vi "RT.vi"() -> ()   [LabVIEW 2013]
uses:
  <vilib>/rvi/interface/nirviOpenFPGA/nirviOpenFPGA.xnode
  <vilib>/rvi/interface/nirviCloseFPGA/nirviCloseFPGA.xnode
  <vilib>/rvi/interface/nirviReadWriteControl/nirviReadWriteControl.xnode
  <vilib>/rvi/interface/Simulation/niFpgaSimulationCallBeginRW.vi
  <vilib>/rvi/errors/niLvFpgaAdjustHostInterfaceError.vi
  <vilib>/Utility/error.llb/Error Cluster From Error Code.vi
  FPGA Bitfiles/AudurLoadControl_FPGATarget_FPGA_+jw7eAiF5hA.lvbitx
  FPGA.vi
  <vilib>/FPGAPlugInAG/cRIO-9082/niLvFpga_Open_cRIO-9082.vi
  <vilib>/rvi/interface/common/dynamic/niFpgaDynamicAddResources.vi
  NiFpgaLv.dll
  <vilib>/FPGAPlugInAG/Dynamic/niLvFpga_Close_Dynamic.vi
panel:
  in  "Alpha":sgl
  in  "Scaling":sgl
  in  "Freq of Osc":sgl
  out "Monitoring Loop Period":u32
  out "Input Selection Loop Period":u32
  in  "Input pick":u16
  # "Input singal picking:\n0 Active Power \n1 Positive seq. volt A1\n2 Positive seq. volt A2\n3 Positive seq. current A1\n4 Positive seq. current A2\n5 Volt angle difference"
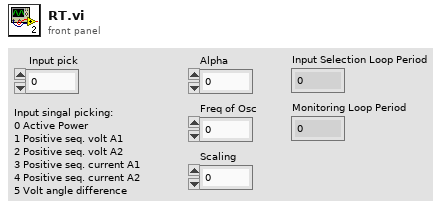
[diagram p1: front panel]
types:
  T1 = cluster{"Parameters":cluster{"Ts":sgl, "kappaav":sgl, "kappaph":sgl, "mu":sgl}}
  T2 = cluster{"Input signal":sgl, "Control signal":sgl, " Empty":sgl, " Empty":sgl}
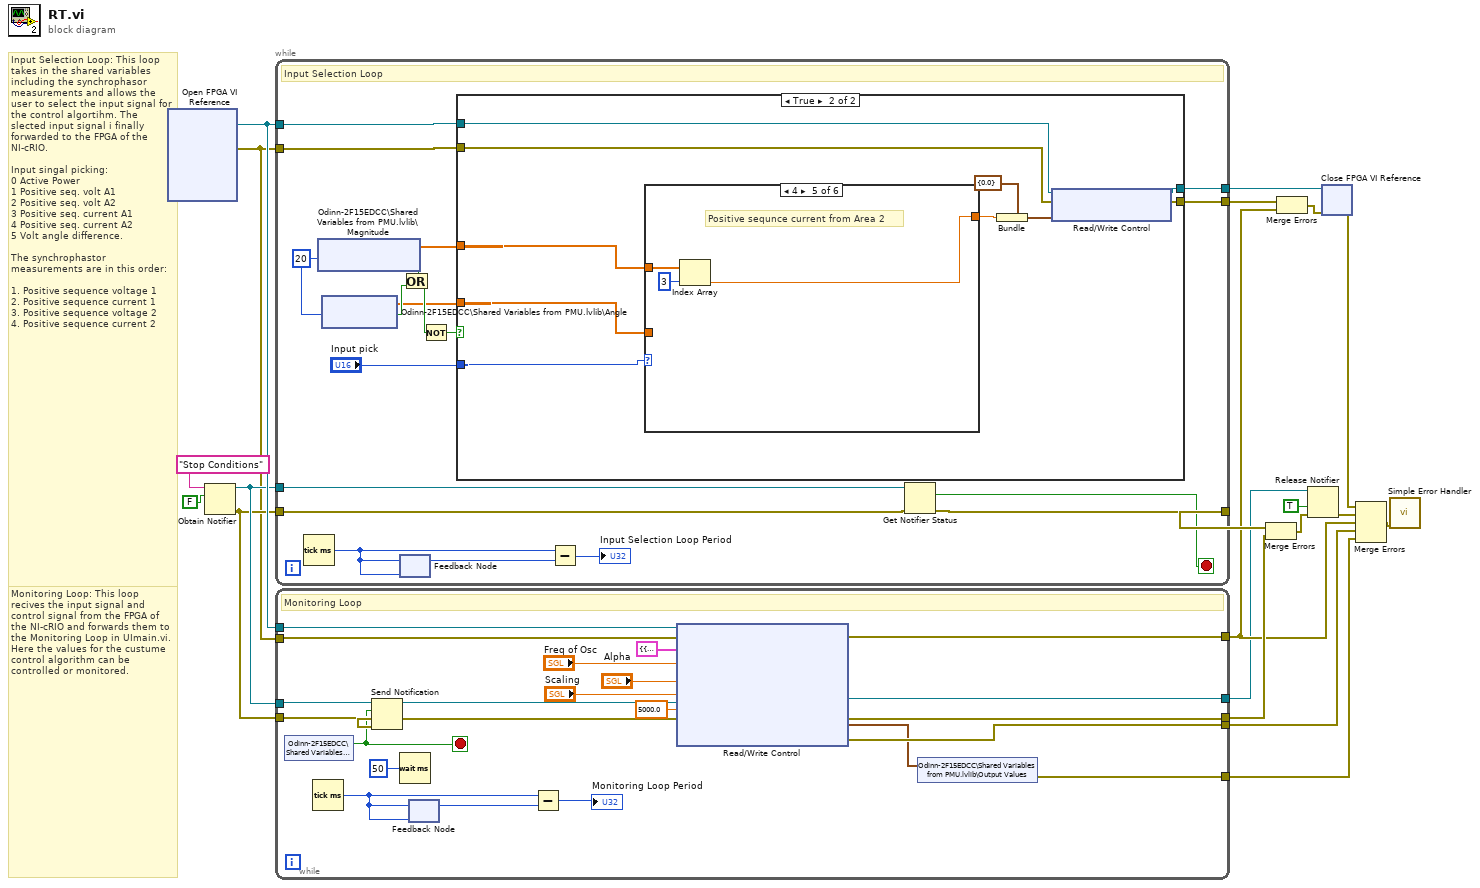
[diagram p0: block diagram]
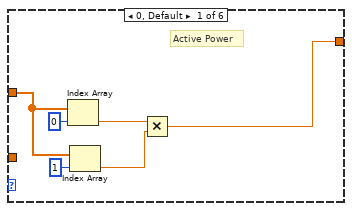
[diagram p3: hidden frame]
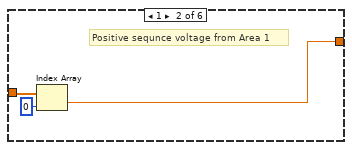
[diagram p4: hidden frame]
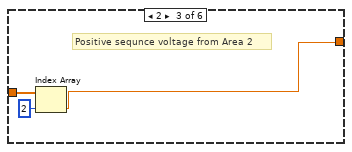
[diagram p5: hidden frame]
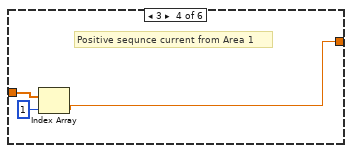
[diagram p6: hidden frame]
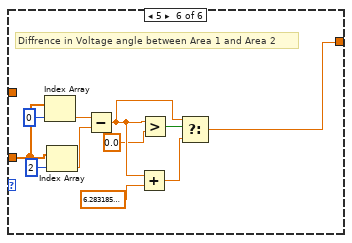
[diagram p7: hidden frame]
diagram:
  # "Monitoring Loop: This loop recives the input signal and control signal from the FPGA of the NI-cRIO and forwards them to the Monitoring Loop in UImain.vi. Here the values for the custume control algorithm can be controlled or monitored."
  # "Input Selection Loop: This loop takes in the shared variables including the synchrophasor measurements and allows the user to select the input signal for the control algortihm. The slected input signal i finally forwarded to the FPGA of the NI-cRIO.\n\nInput singal picking:\n0 Active Power \n1 Positive seq. volt A1\n2 Positive seq. volt A2\n3 Positive seq. current A1\n4 Positive seq. current A2\n5 Volt angle difference.\n\nThe synchrophastor measurements are in this order:\n\n1. Positive sequence voltage 1\n2. Positive sequence current 1\n3. Positive sequence voltage 2\n4. Positive sequence current 2"
  n1 = xnode "Open FPGA VI Reference"() -> ("FPGA VI Reference Out"=w20:refnum<k20>, "error out"=w1:errorcluster)  [unwired: 2 in]
  n2 = Obtain Notifier(name (unnamed)="Stop Conditions", notification data type=FALSE) -> (notifier out=w3:refnum<notifier>, error out=w2:errorcluster)  [unwired: 2 in, 1 out]
  n3 = while {
    tunnel: w20 -> [w35]
    tunnel: w1 -> [w39]
    tunnel: [w38] -> w7
    tunnel: [w32] -> w10
    tunnel: w3 -> [w25]
    tunnel: w2 -> [w24]
    tunnel: [w23] -> w13
    stop <- w22 stop-if-true
    w31 = 20 ("ms timeout (0)")
    # "Input Selection Loop"
    n4 = Tick Count (ms)() -> (millisecond timer value=w37:u32)
    n5 = shared-variable "Odinn-2F15EDCC\\Shared Variables from PMU.lvlib\\Magnitude"(w31) -> (w34:sgl[], w30:bool)  [unwired: 1 in, 1 out]
    n6 = shared-variable "Odinn-2F15EDCC\\Shared Variables from PMU.lvlib\\Angle"(w31) -> (w26:sgl[], w29:bool)  [unwired: 1 in, 1 out]
    n7 = feedback #1(w37) -> (w36:u32)
    n8 = feedback-in #1(w37) -> ()
    n9 = Or(x=w30, y=w29) -> (x .or. y?=w28:bool)
    n10 = Not(x=w28) -> (.not. x?=w33:bool)
    n11 = case shown="True" w33 {
      tunnel: w39 -> [w40 w51]
      tunnel: [w41 w50] -> w38
      tunnel: [w40 w49] -> w32
      tunnel: w35 -> [w41 w48]
      tunnel: w34 -> [_ w43]
      tunnel: "Input pick" -> [_ w47]
      tunnel: w26 -> [_ w42]
      frame False {
      }
      frame True {
        n12 = case shown="4" w47 {
          tunnel: w43 -> [w57 w60 w63 w66 w69 _]
          tunnel: w42 -> [_ _ _ _ _ w80]
          tunnel: [w52 w58 w61 w64 w67 w70] -> w44
          frame 0, Default {
            # "Active Power"
            n13 = Index Array(array=w57, index=0) -> (element=w54:sgl)
            n14 = Index Array(array=w57, index=1) -> (element=w53:sgl)
            n15 = Multiply(x=w54, y=w53) -> (x*y=w52:sgl)
          }
          frame 1 {
            # "Positive sequnce voltage from Area 1"
            n16 = Index Array(array=w60, index=0) -> (element=w58:sgl)
          }
          frame 2 {
            # "Positive sequnce voltage from Area 2"
            n17 = Index Array(array=w63, index=2) -> (element=w61:sgl)
          }
          frame 3 {
            # "Positive sequnce current from Area 1"
            n18 = Index Array(array=w66, index=1) -> (element=w64:sgl)
          }
          frame 4 {
            # "Positive sequnce current from Area 2"
            n19 = Index Array(array=w69, index=3) -> (element=w67:sgl)
          }
          frame 5 {
            # "Diffrence in Voltage angle between Area 1 and Area 2"
            n20 = Index Array(array=w80, index=0) -> (element=w77:sgl)
            n21 = Index Array(array=w80, index=2) -> (element=w76:sgl)
            n22 = Subtract(x=w77, y=w76) -> (x-y=w74:sgl)
            n23 = Add(x=w74, y=sgl 6.2831855) -> (x+y=w73:sgl)
            n24 = Greater?(x=w74, y=sgl 0.0 ("x")) -> (0:w75:bool)
            n25 = Select(t=w74, s=w75, f=w73) -> (s? t:f=w70:sgl)
          }
        }
        n26 = Bundle(cluster=cluster{sgl} {0.0}, w44) -> (w46:cluster{sgl})
        n27 = xnode "Read/Write Control"("FPGA VI Reference In"=w48, "error in"=w51, "PMU measurments"=w46) -> ("FPGA VI Reference Out"=w50:refnum<k20>, "error out"=w49:errorcluster)
      }
    }
    n28 = Subtract(x=w37, y=w36) -> (x-y=→"Input Selection Loop Period":u32)
    n29 = Get Notifier Status(notifier=w25, error in (no error)=w24) -> (current notification=w22:bool, error out=w23:errorcluster)  [unwired: 3 out]
  }
  n30 = while {
    tunnel: w20 -> [w100]
    tunnel: w1 -> [w99]
    tunnel: w3 -> [w89]
    tunnel: w2 -> [w90]
    tunnel: [w94] -> w15
    tunnel: [w93] -> w14
    tunnel: [w92] -> w9
    tunnel: [w91] -> w12
    tunnel: [w88] -> w5
    stop <- w87 stop-if-true
    # "Monitoring Loop"
    n31 = shared-variable "Odinn-2F15EDCC\\Shared Variables from PMU.lvlib\\Stop"() -> (w87:bool)  [unwired: 1 in, 1 out]
    n32 = Tick Count (ms)() -> (millisecond timer value=w98:u32)
    n33 = Send Notification(notification=w87, notifier=w89, error in (no error)=w90) -> (notifier out=w88:refnum<notifier>, error out=w91:errorcluster)
    n34 = Wait (ms)(milliseconds to wait=u32 50) -> ()  [unwired: 1 out]
    n35 = feedback #2(w98) -> (w97:u32)
    n36 = feedback-in #2(w98) -> ()
    n37 = Subtract(x=w98, y=w97) -> (x-y=→"Monitoring Loop Period":u32)
    n38 = xnode "Read/Write Control"("FPGA VI Reference In"=w100, "error in"=w99, "Frequency Estimator Settings"=T1 {"Parameters"={"Ts"=5e-05, "kappaav"=0.625, "kappaph"=0.5762, "mu"=0.7086}}, "Freq of Osc Load"="Freq of Osc", "alpha_Load"="Alpha", "Scaling"="Scaling", "Hold Time"=sgl 5000.0) -> ("error out"=w92:errorcluster, "output cluster"=w85:T2, "FPGA Error Out"=w94:errorcluster)  [unwired: 1 out]
    n39 = shared-variable "Odinn-2F15EDCC\\Shared Variables from PMU.lvlib\\Output Values"(w85) -> (error out=w93:errorcluster)  [unwired: 1 in]
  }
  n40 = Merge Errors(w13, w12) -> (w11:errorcluster)
  n41 = Merge Errors(w10, w9) -> (w8:errorcluster)
  n42 = Release Notifier(notifier=w5, force destroy? (F)=TRUE, error in (no error)=w11) -> (error out=w6:errorcluster)  [unwired: 2 out]
  n43 = xnode "Close FPGA VI Reference"("FPGA VI Reference In"=w7, "error in"=w8) -> ("error out"=w17:errorcluster)
  n44 = Merge Errors(w17, w6, w9, w15, w14) -> (w16:errorcluster)
  n45 = call <vilib>:"Simple Error Handler.vi"("error in (no error)"=w16) -> ()  [unwired: 4 in, 5 out]
